vi "Find diff in axis.vi"(10 "array":dbl[](array[numeric])) -> (2 "x,y2 - x,y1":dbl[](array[numeric]))   [LabVIEW 2016]
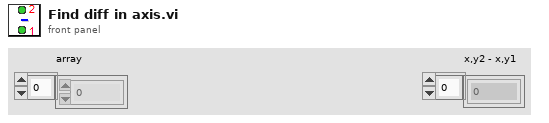
[diagram p1: front panel]
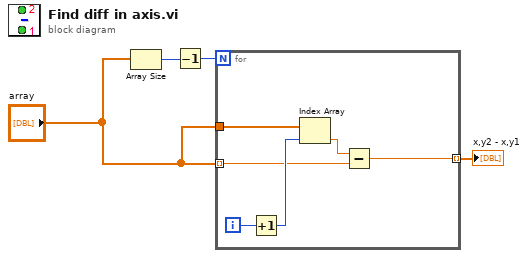
[diagram p0: block diagram]
diagram:
  n1 = Array Size(array="array") -> (size(s)=w4:i32)
  n2 = Decrement(x=w4) -> (x-1=w3:i32)
  n3 = for {
    N: w3 -> [_]
    tunnel: "array" -> [w6] mode=indexing
    tunnel: "array" -> [w10]
    tunnel: [w5] -> w1 mode=indexing
    i -> [w9]
    n4 = Increment(x=w9) -> (x+1=w8:i32)
    n5 = Index Array(array=w10, index=w8) -> (element=w7:dbl)
    n6 = Subtract(x=w7, y=w6) -> (x-y=w5:dbl)
  }
  "x,y2 - x,y1" <- w1
